vi "Read Move Speed.vi"(8 "error in (no error)":errorcluster, 11 "Crosshair Dispense in":refnum<class "Crosshair Dispense.lvclass">) -> (0 "error out":errorcluster, 2 "Move Speed":i32, 3 "Crosshair Dispense out":refnum<class "Crosshair Dispense.lvclass">)   [LabVIEW 2019, in "Crosshair Dispense.lvclass"]
uses:
  Crosshair Dispense.lvclass
  Crosshair Dispense.lvclass/Crosshair Dispense.ctl
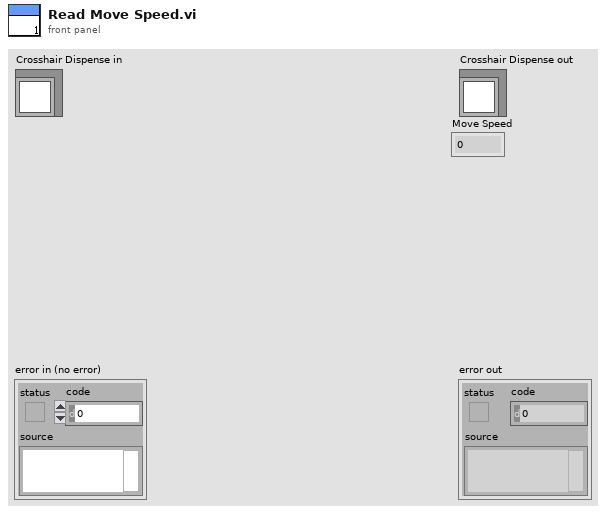
[diagram p1: front panel]
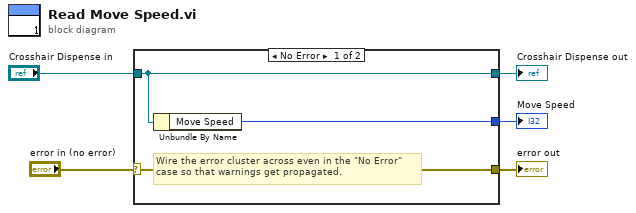
[diagram p0: block diagram]
diagram:
  n1 = case shown="No Error" "error in (no error)" {
    selector: "error in (no error)" -> [w8 w10]
    tunnel: [w8 w10] -> w4
    tunnel: [w7 w9] -> w2
    tunnel: "Crosshair Dispense in" -> [w7 w9]
    tunnel: [w6 _] -> w1
    frame No Error {
      # "Wire the error cluster across even in the \"No Error\"\ncase so that warnings get propagated."
      n2 = Unbundle By Name(w7) -> ("Move Speed"=w6:i32)
    }
    frame Error {
    }
  }
  "error out" <- w4
  "Crosshair Dispense out" <- w2
  "Move Speed" <- w1
